vi "Draw XY Heading.vi"(10 "Length":dbl, 11 "Direction":dbl) -> (3 "Heading Graph":cluster{dbl[], dbl[]})   [LabVIEW 2018]
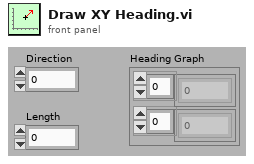
[diagram p1: front panel]
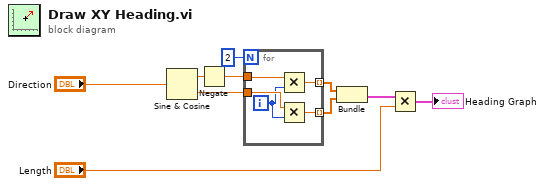
[diagram p0: block diagram]
diagram:
  n1 = Sine & Cosine(0:"Direction") -> (1:w1:dbl, 2:w5:dbl)
  n2 = Negate(x=w1) -> (-x=w4:dbl)
  n3 = for {
    N: 2 -> [_]
    tunnel: w4 -> [w15]
    tunnel: w5 -> [w14]
    tunnel: [w12] -> w6 mode=indexing
    tunnel: [w11] -> w7 mode=indexing
    i -> [w13]
    n4 = Multiply(x=w15, y=w13) -> (x*y=w12:dbl)
    n5 = Multiply(x=w14, y=w13) -> (x*y=w11:dbl)
  }
  n6 = Bundle(w6, w7) -> (w8:cluster{dbl[], dbl[]})  [unwired: 1 out]
  n7 = Multiply(x=w8, y="Length") -> (x*y=→"Heading Graph":cluster{dbl[], dbl[]})
